vi "Active Power-Spectrum Method-v2.vi"() -> ()   [LabVIEW 2014]
uses:
  <vilib>/DAQmx/create/channels.llb/DAQmx Create Channel (AI-Voltage-Basic).vi
  <vilib>/DAQmx/configure/timing.llb/DAQmx Timing (Sample Clock).vi
  <vilib>/DAQmx/read.llb/DAQmx Read (Analog 1D DBL 1Chan NSamp).vi
panel:
  in  "ms to cut at the end (ms)":dbl
  in  "Fs,#points":dbl
  in  "Custum Fs (Hz)":i32
  in  "Sampling Rate (Hz) 2":T1(ring)=enum."16384"
  out "Axis":i32
  out "final Real Current Commanded position (um)":dbl
  out "Real Current Commanded position (um)":dbl format="%0.5f"
  out "Samples per channel":dbl
  out "physical channels":tag
  out "stiffness from diffusion coeff.(pN/nm)":dbl
  in  "Temp (C)":dbl
  out "stiffness from friction coeff.(pN/nm)":dbl format="%#_6f"
  out "Diffusion coefficient, D (V^2/s)":dbl
  out "a1":dbl
  in  "bead height (um)":dbl=1.0
  in  "bead radius (um)":dbl=0.515
  out "Beta (V/um)":dbl
  out "fResponse (Hz)":dbl
  out "Wex":dbl
  out "Wth":dbl
  out "fc":dbl
  out "best fit parameters\n(XX,fc)":dbl[](array[numeric])
  in  "Freq End Cut":dbl
  in  "Freq Strat Cut":dbl
  out "Frequency (Hz)\n0,df, 2df,...(n/2-1)Fs":dbl[](array[numeric])
  out "Avg. PSD":dbl[](array[numeric])
  out "Avg. completed":i32
  in  "Tab Control":enum32{"Page 1", "Page 3", "Page 2"}(tab)
  out "XY Graph":T2(graph)
  out "Waveform Graph":dbl[](graph)
  out "XY Graph 2":T3(graph)
  in  "Cycles to average":i32=30
  out "Sampling Rate (Hz)":i32=32000
  out "Need time (s)":dbl format="%.5f"
  in  "Amplitude, A (nm)":dbl=200.0
  in  "f_drive (Hz)":dbl=30.0
  in  "Axis (Enum)":enum16{"x", "y", "z"}(ring)
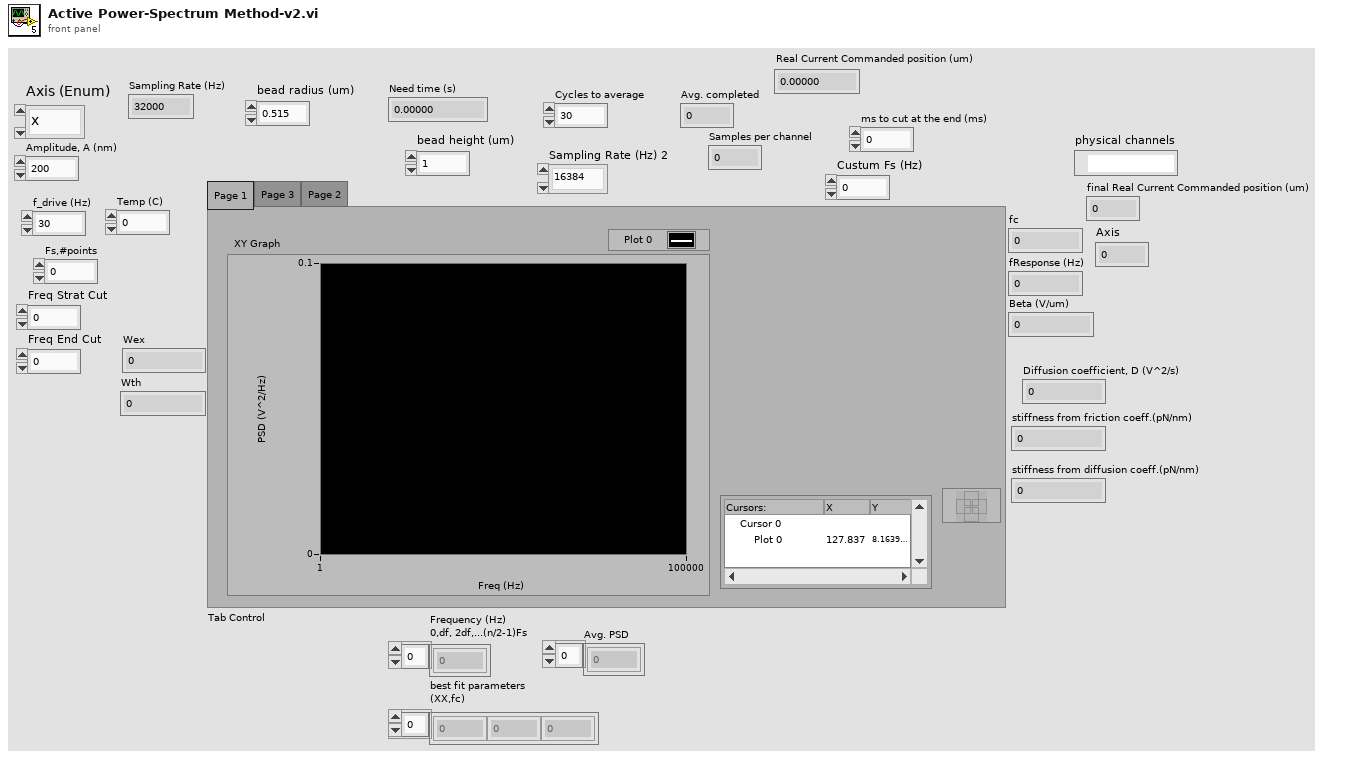
[diagram p1: front panel]
types:
  T1 = enum16{"custum", "16384", "32768", "65536", "131072"}
  T2 = cluster{"Frequency (Hz)\n0,df, 2df,...(n/2-1)Fs":dbl[], dbl[]}
  T3 = cluster{"Frequency (Hz)\n0,df, 2df,...(n/2-1)Fs":dbl[], dbl[]}[]
  T4 = cluster{"Freq Cut":dbl[], "best nonlinear fit PSD":dbl[]}
  T5 = cluster{"Frequency (Hz)\n0,df, 2df,...(n/2-1)Fs":dbl[], "best nonlinear fit PSD":dbl[]}[]
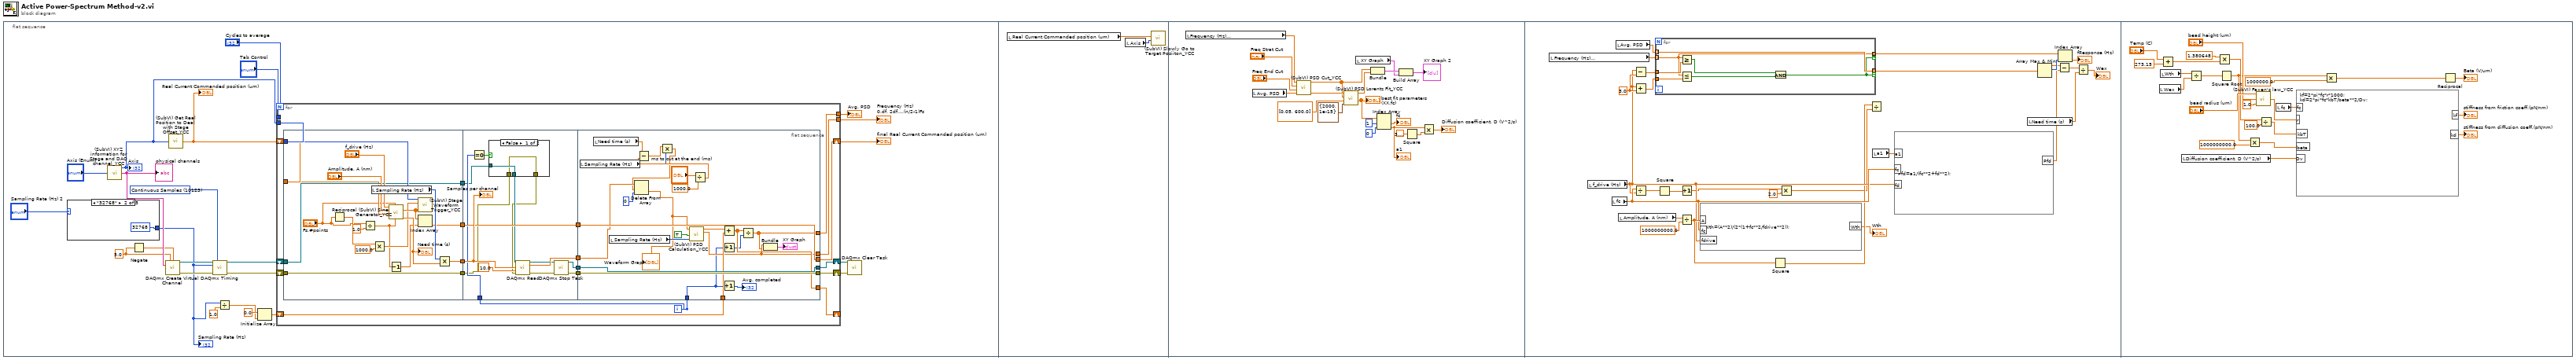
[diagram p0: block diagram]
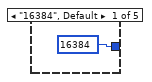
[diagram p2: hidden frame]
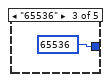
[diagram p3: hidden frame]
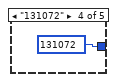
[diagram p4: hidden frame]
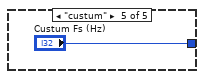
[diagram p5: hidden frame]
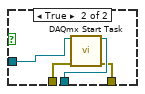
[diagram p6: hidden frame]
diagram:
  n1 = flat-sequence {
    frame #0 {
      w17 = 10123 items=["Finite Samples"=10178, "Continuous Samples"=10123, "Hardware Timed Single Point"=12522] ("sample mode")
      w21 = 5.0 ("maximum value")
      n2 = case shown="\"32768\"" "Sampling Rate (Hz) 2" {
        tunnel: [16384 32768 65536 131072 "Custum Fs (Hz)"] -> w5
        frame "16384", Default {
        }
        frame "32768" {
        }
        frame "65536" {
        }
        frame "131072" {
        }
        frame "custum" {
        }
      }
      "Sampling Rate (Hz)" <- w5
      n3 = call "(SubVI) XYZ information for Stage and DAQ channel_YCC.vi"("Axis  (Enum)"="Axis (Enum)") -> ("physical channels"=w22:tag, "Axis"=w14:i32)  [unwired: 3 in]
      "physical channels" <- w22
      "Axis" <- w14
      n4 = Negate(x=w21) -> (-x=w20:dbl)
      n5 = call-poly <vilib>:"DAQmx Create Virtual Channel.vi"("maximum value"=w21, "minimum value"=w20, "physical channels"=w22) -> ("task out"=w19:refnum<k21>, "error out"=w18:errorcluster)  [unwired: 11 in]
      n6 = call "(SubVI) Get Real Position to Deal with Stage Offset_YCC.vi"("Axis"=w14) -> ("Real Current Commanded position (um)"=w13:dbl)  [unwired: 3 in, 1 out]
      "Real Current Commanded position (um)" <- w13
      n7 = call-poly <vilib>:"DAQmx Timing.vi"("task/channels in"=w19, "sample mode"=w17, "rate"=w5, "error in"=w18) -> ("task out"=w2:refnum<k21>, "error out"=w1:errorcluster)  [unwired: 3 in, 7 out]
      n8 = Divide(x=w5, y=1.0) -> (x/y=w4:dbl)
      n9 = Initialize Array(0.0 ("element"), w4) -> (w10:dbl[])
      n10 = for {
        N: "Cycles to average" -> [_]
        tunnel: w14 -> [w48]
        shift-right: [w47] -> w16
        shift-left: w2 -> [w44]
        shift-right: [w46] -> w15
        shift-left: w1 -> [w42]
        shift-right: [w37] -> w7
        shift-left: w13 -> [w38]
        tunnel: "Tab Control" -> [_]
        shift-right: [w33] -> _
        shift-left: w10 -> [w34]
        tunnel: [w32] -> w9
        tunnel: [w31] -> w8
        i -> [w30]
        n11 = flat-sequence {
          tunnel: w48 -> [w65]
          tunnel: [w63] -> w49
          tunnel: [w61] -> w45
          tunnel: w44 -> [w61]
          tunnel: [w60] -> w43
          tunnel: w42 -> [w60]
          tunnel: w38 -> [w59]
          tunnel: [w56] -> w35
          tunnel: w43 -> [w70]
          tunnel: w45 -> [w71]
          tunnel: w49 -> [w80]
          tunnel: [w81] -> w41
          tunnel: [w75] -> w40
          tunnel: [w74] -> w39
          tunnel: [w78] -> w36
          tunnel: w35 -> [w78]
          tunnel: w30 -> [w72]
          tunnel: [w110] -> w46
          tunnel: [w111] -> w47
          tunnel: w41 -> [w97]
          tunnel: w40 -> [w111]
          tunnel: w39 -> [w110]
          tunnel: [w107] -> w37
          tunnel: w36 -> [w107]
          tunnel: w34 -> [w106]
          tunnel: [w103] -> w33
          tunnel: w30 -> [w98]
          tunnel: [w101] -> w32
          tunnel: [w100] -> w31
          frame #0 {
            n12 = Reciprocal(x="Fs,#points") -> (1/x=w52:dbl)
            n13 = Divide(x="Fs,#points", y=1.0) -> (x/y=w50:dbl)
            n14 = local read "Sampling Rate (Hz)"() -> (w64:i32)
            n15 = Multiply(x=w52, y=1000.0) -> (x*y=w54:dbl)
            n16 = call "(SubVI) Sine Generator_YCC.vi"("Points to be generated"=w50, "fs (Hz)"="Fs,#points", "initial position (um)"=w59, "Amplitude, A (nm)"="Amplitude, A (nm)", "f_drive (Hz)"="f_drive (Hz)") -> ("Total Need time (s)"=w62:dbl, "Position Array (um)"=w57:dbl[])  [unwired: 1 in, 2 out]
            "Need time (s)" <- w62
            n17 = Decrement(x=w50) -> (x-1=w58:dbl)
            n18 = call "(SubVI) Stage Waveform Trigger_YCC.vi"("Position Array (um)"=w57, "milliseconds to wait"=w54, "axis"=w65) -> ()  [unwired: 5 in]
            n19 = Index Array(array=w57, index=w58) -> (element=w56:dbl)
            n20 = Multiply(x=w64, y=w62) -> (x*y=w63:dbl)
          }
          frame #1 {
            n21 = Equal To 0?(x=w72) -> (x = 0?=w73:bool)
            n22 = case shown="False" w73 {
              tunnel: w71 -> [w83 w87]
              tunnel: w70 -> [w82 w86]
              tunnel: [w83 w85] -> w69
              tunnel: [w82 w84] -> w68
              frame False {
              }
              frame True {
                n23 = call <vilib>:"DAQmx Start Task.vi"("task/channels in"=w87, "error in"=w86) -> ("task out"=w85:refnum<k21>, "error out"=w84:errorcluster)  [unwired: 12 out]
              }
            }
            n24 = call-poly <vilib>:"DAQmx Read.vi"("task/channels in"=w69, "number of samples per channel"=w80, "timeout"=10.0, "error in"=w68) -> ("task out"=w77:refnum<k21>, "data"=w81:dbl[], "error out"=w76:errorcluster)  [unwired: 9 in]
            n25 = call <vilib>:"DAQmx Stop Task.vi"("task/channels in"=w77, "error in"=w76) -> ("task out"=w75:refnum<k21>, "error out"=w74:errorcluster)  [unwired: 12 in]
            "Samples per channel" <- w80
          }
          frame #2 {
            n26 = local read "Sampling Rate (Hz)"() -> (w90:i32)
            n27 = local read "Need time (s)"() -> (w92:dbl)
            n28 = local read "Sampling Rate (Hz)"() -> (w108:i32)
            n29 = Divide(x="ms to cut at the end (ms)", y=1000.0) -> (x/y=w93:dbl)
            n30 = Subtract(x=w92, y=w93) -> (x-y=w91:dbl)
            n31 = Multiply(x=w91, y=w90) -> (x*y=w89:dbl)
            n32 = Delete From Array(array=w97, length=w89, index=0) -> (deleted portion=w88:dbl[])  [unwired: 1 out]
            "Waveform Graph" <- w88
            n33 = call "(SubVI) PSD Calculation_YCC.vi"("sampling frequency (Hz)"=w108, "T=NI made PSD\nF=YCC made PSD"=TRUE ("T=NI made PSD\nF=YCC made PSD"), "QPD data"=w88) -> ("Frequency (Hz)\n0,df, 2df,...(n/2-1)Fs"=w101:dbl[], "Power Spectrum (V^2 rms) (V^2/Hz)"=w105:dbl[])  [unwired: 3 in]
            n34 = Add(x=w105, y=w106) -> (x+y=w103:dbl[])
            n35 = Increment(x=w98) -> (x+1=w102:i32)
            n36 = Increment(x=w98) -> (x+1=→"Avg. completed":i32)
            n37 = Divide(x=w103, y=w102) -> (x/y=w100:dbl[])
            n38 = Bundle("Frequency (Hz)\n0,df, 2df,...(n/2-1)Fs"=w101, w100) -> (→"XY Graph":T2)  [unwired: 1 in]
          }
        }
      }
      "Avg. PSD" <- w8
      "Frequency (Hz)\n0,df, 2df,...(n/2-1)Fs" <- w9
      "final Real Current Commanded position (um)" <- w7
      n39 = call <vilib>:"DAQmx Clear Task.vi"("task in"=w16, "error in"=w15) -> ()  [unwired: 13 in, 1 out]
    }
    frame #1 {
      n40 = local read "Real Current Commanded position (um)"() -> (w113:dbl)
      n41 = local read "Axis"() -> (w112:i32)
      n42 = call "(SubVI) Slowly Go to Target Posiiton_YCC.vi"("axis"=w112, "Target position (um)"=w113) -> ()  [unwired: 2 in, 4 out]
    }
    frame #2 {
      n43 = local read "Frequency (Hz)\n0,df, 2df,...(n/2-1)Fs"() -> (w116:dbl[])
      n44 = local read "Avg. PSD"() -> (w115:dbl[])
      n45 = call "(SubVI) PSD Cut_YCC.vi"("PSD"=w115, "Freq End Cut"="Freq End Cut", "Freq Strat Cut"="Freq Strat Cut", "Frequency (Hz)"=w116) -> ("PSD Cut"=w131:dbl[], "Freq Cut"=w128:dbl[])  [unwired: 2 in]
      n46 = call "(SubVI) PSD Lorentz Fit_YCC.vi"("termination"=cluster{"max iteration":i32, "tolerance":dbl} {"max iteration"=2000, "tolerance"=1e-15}, "initial parameters"=dbl[] [0.05, 600.0], "Frequency (Hz)"=w128, "PSD (Vrms^2)"=w131) -> ("best fit parameters"=w124:dbl[], "best nonlinear fit PSD"=w127:dbl[])  [unwired: 2 in]
      "best fit parameters\n(XX,fc)" <- w124
      n47 = local read "XY Graph"() -> (w125:T2)
      n48 = Bundle("Freq Cut"=w128, "best nonlinear fit PSD"=w127) -> (w126:T4)  [unwired: 1 in]
      n49 = Index Array(array=w124, index #1=1 ("index"), index #2=0 ("index")) -> (element #1=→"fc":dbl, element #2=w118:dbl)
      "a1" <- w118
      n50 = Build Array(w126, w125) -> (→"XY Graph 2":T5)
      n51 = Square(x=3.141592653589793) -> (x^2=w119:dbl)
      n52 = Multiply(x=w118, y=w119) -> (x*y=→"Diffusion coefficient, D (V^2/s)":dbl)
    }
    frame #3 {
      w158 = 3.0 ("y")
      n53 = local read "Frequency (Hz)\n0,df, 2df,...(n/2-1)Fs"() -> (w159:dbl[])
      n54 = local read "f_drive (Hz)"() -> (w141:dbl)
      n55 = local read "fc"() -> (w142:dbl)
      n56 = local read "Avg. PSD"() -> (w160:dbl[])
      n57 = local read "Amplitude, A (nm)"() -> (w145:dbl)
      n58 = Subtract(x=w141, y=w158) -> (x-y=w157:dbl)
      n59 = Add(x=w141, y=w158) -> (x+y=w156:dbl)
      n60 = Divide(x=w142, y=w141) -> (x/y=w140:dbl)
      n61 = for {
        tunnel: [w167] -> w155 mode=indexing if=w161
        tunnel: w160 -> [w167] mode=indexing
        tunnel: [w165] -> w154 mode=indexing if=w161
        tunnel: w159 -> [w165] mode=indexing
        tunnel: w157 -> [w166]
        tunnel: w156 -> [w164]
        n62 = Greater Or Equal?(x=w165, y=w166) -> (x >= y?=w163:bool)
        n63 = Less Or Equal?(x=w165, y=w164) -> (x <= y?=w162:bool)
        n64 = And(x=w163, y=w162) -> (x .and. y?=w161:bool)
      }
      n65 = Square(x=w140) -> (x^2=w139:dbl)
      n66 = Increment(x=w139) -> (x+1=w138:dbl)
      n67 = Divide(x=w145, y=1000000000.0) -> (x/y=w143:dbl)
      n68 = formula code="Wth=(A**2)/(2*(1+fc**2/fdrive**2));"("A"=w143, "fc"=w142, "fdrive"=w141) -> ("Wth"=→"Wth":dbl)
      n69 = Square(x=w143) -> (x^2=w136:dbl)
      n70 = Multiply(x=w138, y=2.0) -> (x*y=w135:dbl)
      n71 = Divide(x=w136, y=w135) -> ()  [unwired: 1 out]
      n72 = local read "a1"() -> (w151:dbl)
      n73 = formula code="Pfd=a1/(fc**2+fd**2);"("a1"=w151, "fc"=w142, "fd"=w141) -> ("Pfd"=w149:dbl)
      n74 = local read "Need time (s)"() -> (w147:dbl)
      n75 = Array Max & Min(array=w155) -> (max value=w150:dbl, max index (indices)=w153:i32)  [unwired: 2 out]
      n76 = Subtract(x=w150, y=w149) -> (x-y=w148:dbl)
      n77 = Index Array(array=w154, index=w153) -> (element=→"fResponse (Hz)":dbl)
      n78 = Divide(x=w148, y=w147) -> (x/y=→"Wex":dbl)
    }
    frame #4 {
      n79 = local read "Wex"() -> (w190:dbl)
      n80 = local read "Wth"() -> (w191:dbl)
      n81 = Add(x="Temp (C)", y=273.15) -> (x+y=w181:dbl)
      n82 = local read "Diffusion coefficient, D (V^2/s)"() -> (w174:dbl)
      n83 = Divide(x=w191, y=w190) -> (x/y=w171:dbl)
      n84 = Multiply(x=1.380648, y=w181) -> (x*y=w180:dbl)
      n85 = Square Root(x=w171) -> (sqrt(x)=w170:dbl)
      n86 = Multiply(x=w170, y=1000000000.0) -> (x*y=w168:dbl)
      n87 = call "(SubVI) Faxen's law_YCC.vi"("viscosity (cP)"=1.0, "bead height (um)"="bead height (um)", "bead radius (um)"="bead radius (um)") -> ("Faxen's law of friction coefficient (N/(m/s))"=w176:dbl)  [unwired: 2 in]
      n88 = Divide(x=w180, y=100.0) -> (x/y=w178:dbl)
      n89 = local read "fc"() -> (w177:dbl)
      n90 = formula code="kf=2*pi*fc*r*1000;\nkd=2*pi*fc*kbT/beta**2/Dv;"("fc"=w177, "r"=w176, "kbT"=w178, "beta"=w168, "Dv"=w174) -> ("kf"=→"stiffness from friction coeff.(pN/nm)":dbl, "kd"=→"stiffness from diffusion coeff.(pN/nm)":dbl)
      n91 = Multiply(x=w170, y=1000000.0) -> (x*y=w175:dbl)
      n92 = Reciprocal(x=w175) -> (1/x=→"Beta (V/um)":dbl)
    }
  }
